vi "Disable Keys.vi"(0 "Boolean in":refnum<vi>, 1 "Bool Refnum 6":refnum<vi>, 2 "Bool Refnum 4":refnum<vi>, 3 "Bool Refnum 7":refnum<vi>, 4 "Bool Refnum 9":refnum<vi>, 5 "Bool Refnum 2":refnum<vi>, 6 "Bool Refnum 8":refnum<vi>, 7 "Bool Refnum 3":refnum<vi>) -> ()   [LabVIEW 2019]
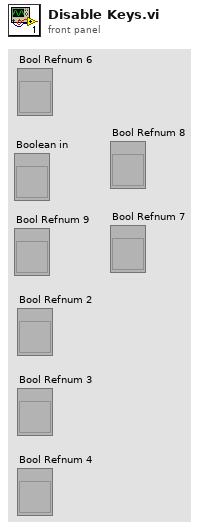
[diagram p1: front panel]
types:
  T1 = enum8{"Enabled", "Disabled", "Disabled and Grayed Out"}
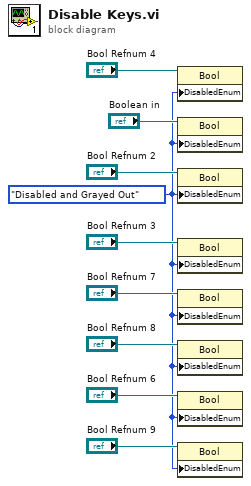
[diagram p0: block diagram]
diagram:
  w1 = T1."Disabled and Grayed Out" ("Disabled")
  n1 = property on="Property Node" class="Bool"(reference="Bool Refnum 4", "DisabledEnum"=w1) -> ()  [unwired: 1 in, 2 out]
  n2 = property on="Property Node" class="Bool"(reference="Boolean in", "DisabledEnum"=w1) -> ()  [unwired: 1 in, 2 out]
  n3 = property on="Property Node" class="Bool"(reference="Bool Refnum 2", "DisabledEnum"=w1) -> ()  [unwired: 1 in, 2 out]
  n4 = property on="Property Node" class="Bool"(reference="Bool Refnum 3", "DisabledEnum"=w1) -> ()  [unwired: 1 in, 2 out]
  n5 = property on="Property Node" class="Bool"(reference="Bool Refnum 7", "DisabledEnum"=w1) -> ()  [unwired: 1 in, 2 out]
  n6 = property on="Property Node" class="Bool"(reference="Bool Refnum 8", "DisabledEnum"=w1) -> ()  [unwired: 1 in, 2 out]
  n7 = property on="Property Node" class="Bool"(reference="Bool Refnum 6", "DisabledEnum"=w1) -> ()  [unwired: 1 in, 2 out]
  n8 = property on="Property Node" class="Bool"(reference="Bool Refnum 9", "DisabledEnum"=w1) -> ()  [unwired: 1 in, 2 out]
